vi "TrimSpaceColRow.vi"(11 "Array in":string[][](array[string])) -> (3 "Array out":string[][](array[string]))   [LabVIEW 2014]
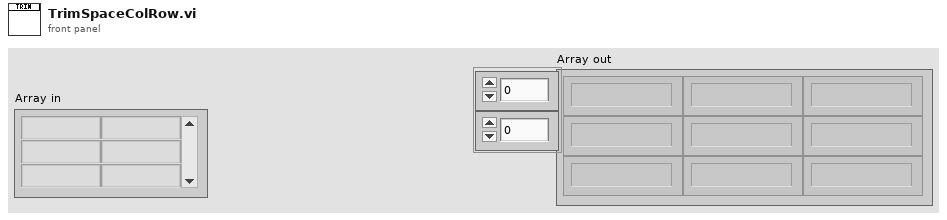
[diagram p1: front panel]
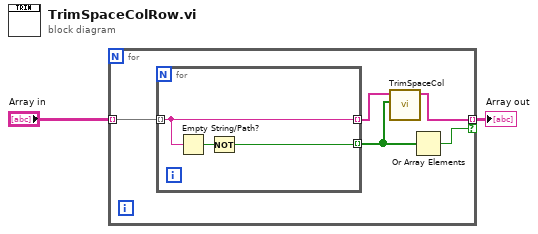
[diagram p0: block diagram]
diagram:
  n1 = for {
    tunnel: "Array in" -> [w7] mode=indexing
    tunnel: [w3] -> w1 mode=indexing if=w6
    n2 = for {
      tunnel: w7 -> [w10] mode=indexing
      tunnel: [w10] -> w5 mode=indexing
      tunnel: [w9] -> w4 mode=indexing
      n3 = Empty String/Path?(string/path=w10) -> (empty?=w8:bool)
      n4 = Not(x=w8) -> (.not. x?=w9:bool)
    }
    n5 = call "TrimSpaceCol.vi"("Bool Array"=w4, "Str Array"=w5) -> ("Array out"=w3:string[])  [unwired: 8 in, 1 out]
    n6 = Or Array Elements(Boolean array=w4) -> (logical OR=w6:bool)
  }
  "Array out" <- w1
